vi "get one frame - subvi.vi"(8 "error in":errorcluster, 9 "Image Height":i32, 10 "Image Width":i32, 11 "Image In":T1) -> (0 "error out":errorcluster, 3 "Image Out":T1)   [LabVIEW 2014]
uses:
  lib/Andorlib/atmcd32d.lvlib
  <vilib>/vision/Image Controls.llb/IMAQ Image.ctl
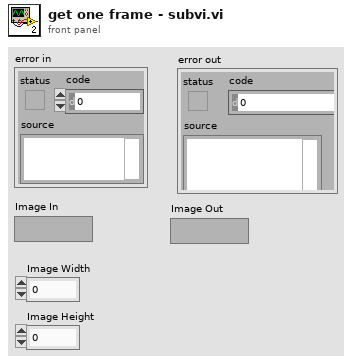
[diagram p1: front panel]
types:
  T1 = typedef "IMAQ Image.ctl" = refnum<image>
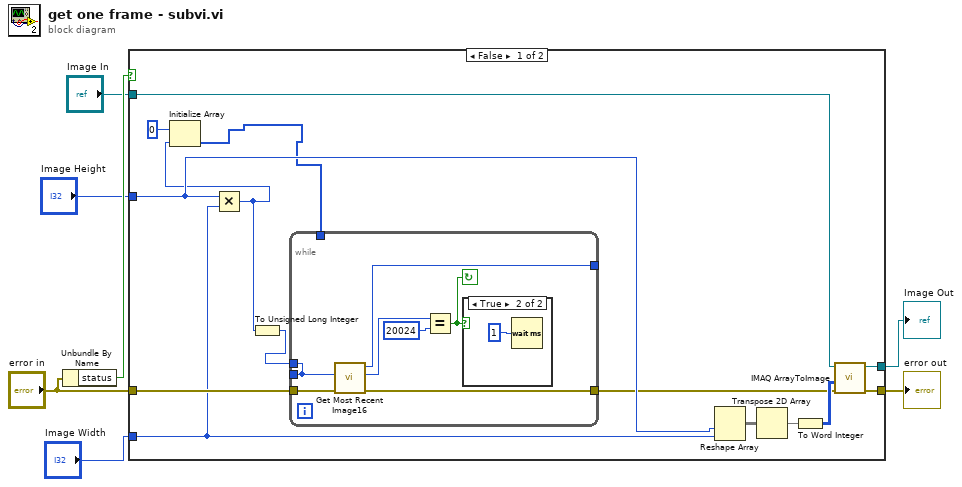
[diagram p0: block diagram]
diagram:
  n1 = Unbundle By Name("error in") -> ("status"=w7:bool)
  n2 = case shown="False" w7 {
    tunnel: "error in" -> [w21 w31]
    tunnel: [w16 w31] -> w2
    tunnel: "Image Height" -> [w20 _]
    tunnel: "Image Width" -> [w19 _]
    tunnel: "Image In" -> [w15 w30]
    tunnel: [w14 w30] -> w1
    frame False {
      n3 = Multiply(x=w20, y=w19) -> (x*y=w12:i32)
      n4 = Initialize Array "Initialize Array"(u16 0, w12) -> (w10:u16[])
      n5 = To Unsigned Long Integer(number=w12) -> (unsigned 32bit integer=w8:u32)
      n6 = while {
        tunnel: [w22] -> _
        tunnel: [w23] -> _
        tunnel: w21 -> [w25]
        tunnel: [w26] -> w9
        tunnel: w10 -> [_]
        tunnel: w8 -> [w22]
        stop <- w27 continue-if-true
        n7 = call <userlib>:"Get Most Recent Image16.vi"("error in (no error)"=w25, "size"=w22) -> ("error out"=w26:errorcluster, "function return"=w24:u32, "arr out"=w23:u16)  [unwired: 7 in]
        n8 = Equal?(x=w24, y=u32 20024) -> (x = y?=w27:bool)
        n9 = case shown="True" w27 {
          frame False {
          }
          frame True {
            n10 = Wait (ms)(milliseconds to wait=u32 1) -> ()  [unwired: 1 out]
          }
        }
      }
      n11 = Reshape Array(w20, w19) -> (w18:void[][])  [unwired: 1 in]
      n12 = Transpose 2D Array(2D array=w18) -> (transposed array=w17:void[][])
      n13 = To Word Integer(number=w17) -> (16bit integer=w13:i16[][])
      n14 = call "IMAQ ArrayToImage"("error in (no error)"=w9, "Image Pixels (I16)"=w13, "Image"=w15) -> ("error out"=w16:errorcluster, "Image Out"=w14:T1)  [unwired: 3 in, 4 out]
    }
    frame True {
    }
  }
  "error out" <- w2
  "Image Out" <- w1
